vi "Periodic Tasks.vi"(8 "error in":errorcluster) -> ()   [LabVIEW 2014]
doc: "This VI runs in parallel to other tasks. It can contain as many user-defined periodic loops as you need. These can carry out PID or other sorts of timed response."
uses:
  <vilib>/Rock Robotics/WPI/Joystick/WPI_JoystickGetSetRefNum.vi
  <vilib>/Rock Robotics/WPI/RobotDrive/WPI_RobotDriveGetSetRefNum.vi
  Robot Global Data.vi
  <vilib>/Rock Robotics/WPI/RobotDrive/WPI_RobotDriveMecanumDrive_Cartesian.vi
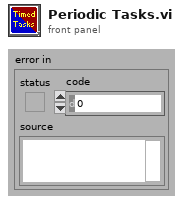
[diagram p1: front panel]
types:
  T1 = typedef "WPI_JoystickDevRef.ctl" = cluster{"Device":T2}
  T2 = typedef "WPI_JoystickDeviceEnum.ctl" = enum16{"USB 0", "USB 1", "USB 2", "USB 3", "USB 4", "USB 5"}
  T3 = typedef "WPI_RobotDriveDevRef.ctl" = cluster{"DevStatus":errorcluster, "Motors[]":T4[], "Square Inputs":bool, "Max Output":dbl}
  T4 = typedef "WPI_MotorControlDeviceRef.ctl" = cluster{"DeviceStatus":errorcluster, "Type":T5, "PWM":cluster{"Controller":T6, "PWM Channel":T7, "DeadBand":T8}, "CAN":cluster{"Device Number":u8, "Control Mode":T9, "Semaphore":T10, "Max Vout":dbl, "TalonSRX Control Mode":T11}, "Invert":bool, "TransformRef":T12, "InvTransformRef":T12}
  T5 = typedef "WPI_MotorControlType.ctl" = enum16{"PWM", "CAN", "CANTalonSRX"}
  T6 = typedef "FPGA_TypedefDigitalModule.ctl" = enum16{"Controller 1"}
  T7 = typedef "FPGA_DIOPWMChannel.ctl" = enum8{"PWM 0", "PWM 1", "PWM 2", "PWM 3", "PWM 4", "PWM 5", "PWM 6", "PWM 7", "PWM 8", "PWM 9", "PWM MXP 0", "PWM MXP 1", "PWM MXP 2", "PWM MXP 3", "PWM MXP 4", "PWM MXP 5", "PWM MXP 6", "PWM MXP 7", "PWM MXP 8", "PWM MXP 9", "Invalid"}
  T8 = typedef "WPI_PWMDeadband.ctl" = cluster{"Name":string, "maxPositivePwm":i32, "minPositivePwm":i32, "centerPwm":i32, "maxNegativePwm":i32, "minNegativePwm":i32, "angularRange":u16}
  T9 = typedef "WPI_CANJaguar_ControlMode.ctl" = enum8{"Percent VBus", "Current", "Speed", "Position", "Voltage"}
  T10 = typedef "Semaphore RefNum" = refnum<k1>
  T11 = typedef "WPI_CANTalonSRX_APIControlMode.ctl" = enum8{"Percent VBus", "Speed", "Position", "Slave", "Unchanged / Invalid"}
  T12 = typedef "WPI_PWMTransform_ConPane.ctl" = refnum<vi>
  T13 = cluster{"JoystickDevRef":T1, "RobotDriveDevRef":T3}
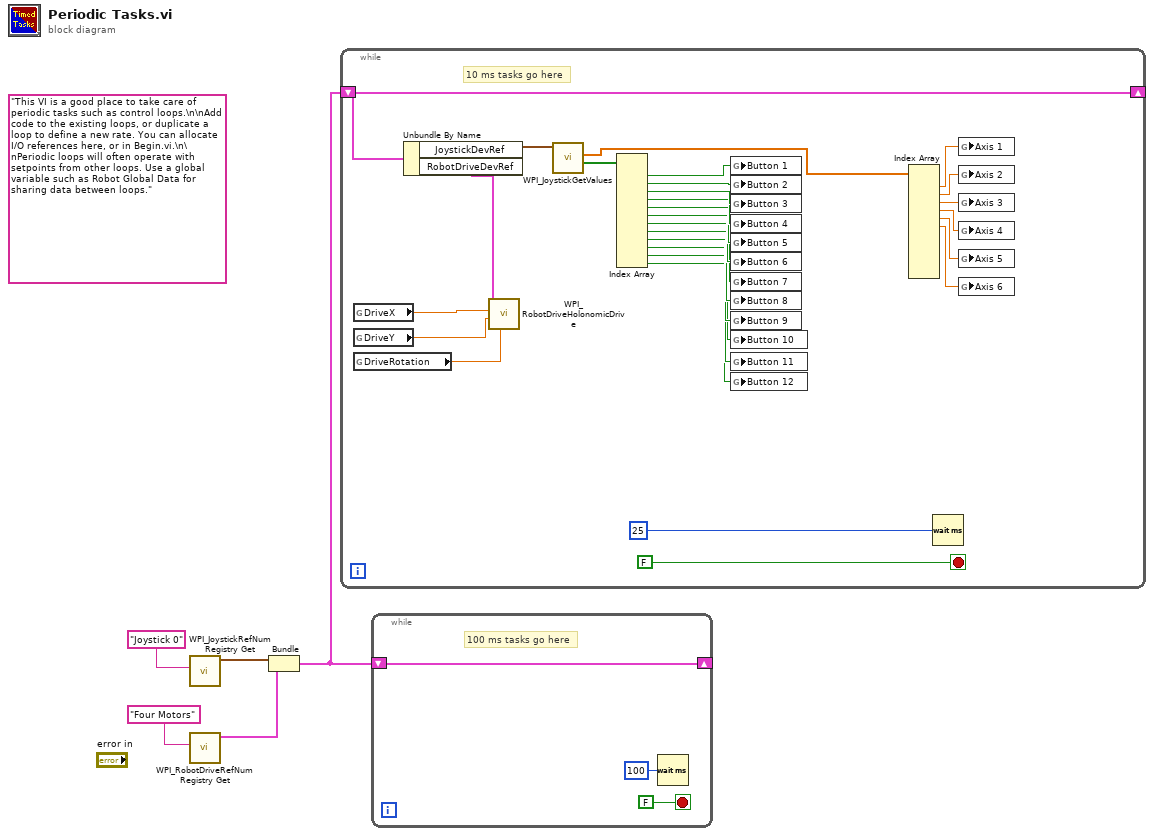
[diagram p0: block diagram]
diagram:
  (unwired) "This VI is a good place to take care of periodic tasks such as control loops.\n\nAdd code to the existing loops, or duplicate a loop to define a new rate. You can allocate I/O references here, or in Begin.vi.\n\nPeriodic loops will often operate with setpoints from other loops. Use a global variable such as Robot Global Data for sharing data between loops."
  n1 = call <vilib>:"WPI_JoystickRefNum Registry Get.vi"("refnum name"="Joystick 0") -> ("JoystickDevRef"=w3:T1)  [unwired: 1 in, 9 out]
  n2 = call <vilib>:"WPI_RobotDriveRefNum Registry Get.vi"("refnum name"="Four Motors") -> ("RobotDriveDevRef"=w2:T3)  [unwired: 1 in, 9 out]
  n3 = Bundle("JoystickDevRef"=w3, "RobotDriveDevRef"=w2) -> (w1:T13)  [unwired: 1 out]
  n4 = while {
    shift-right: [w31] -> _
    shift-left: w1 -> [w31]
    stop <- FALSE stop-if-true
    # "10 ms tasks go here"
    n5 = global read "Robot Global Data.vi" "DriveX"() -> (w8:dbl)
    n6 = global read "Robot Global Data.vi" "DriveY"() -> (w7:dbl)
    n7 = global read "Robot Global Data.vi" "DriveRotation"() -> (w6:dbl)
    n8 = Unbundle By Name(w31) -> ("JoystickDevRef"=w30:T1, "RobotDriveDevRef"=w9:T3)
    n9 = call-poly <vilib>:"WPI_RobotDriveHolonomicDrive.vi"("Rotation"=w6, "Y"=w7, "X"=w8, "RobotDriveDevRef"=w9) -> ()  [unwired: 5 in, 3 out]
    n10 = call <vilib>:"WPI_JoystickGetValues.vi"("JoystickDevRef"=w30) -> ("Buttons"=w29:bool[], "Axes"=w10:dbl[])  [unwired: 6 in, 3 out]
    n11 = Index Array(array=w29) -> (element #1=w28:bool, element #2=w27:bool, element #3=w26:bool, element #4=w25:bool, element #5=w24:bool, element #6=w23:bool, element #7=w22:bool, element #8=w21:bool, element #9=w20:bool, element #10=w19:bool, element #11=w18:bool, element #12=w17:bool)  [unwired: 12 in]
    n12 = global write "Robot Global Data.vi" "Button 1"(w28) -> ()
    n13 = global write "Robot Global Data.vi" "Button 2"(w27) -> ()
    n14 = global write "Robot Global Data.vi" "Button 3"(w26) -> ()
    n15 = global write "Robot Global Data.vi" "Button 4"(w25) -> ()
    n16 = global write "Robot Global Data.vi" "Button 5"(w24) -> ()
    n17 = global write "Robot Global Data.vi" "Button 6"(w23) -> ()
    n18 = global write "Robot Global Data.vi" "Button 7"(w22) -> ()
    n19 = global write "Robot Global Data.vi" "Button 8"(w21) -> ()
    n20 = global write "Robot Global Data.vi" "Button 9"(w20) -> ()
    n21 = global write "Robot Global Data.vi" "Button 10"(w19) -> ()
    n22 = global write "Robot Global Data.vi" "Button 11"(w18) -> ()
    n23 = global write "Robot Global Data.vi" "Button 12"(w17) -> ()
    n24 = Index Array(array=w10) -> (element #1=w16:dbl, element #2=w15:dbl, element #3=w14:dbl, element #4=w13:dbl, element #5=w12:dbl, element #6=w11:dbl)  [unwired: 12 in, 6 out]
    n25 = Wait (ms)(milliseconds to wait=u32 25) -> ()  [unwired: 1 out]
    n26 = global write "Robot Global Data.vi" "Axis 1"(w16) -> ()
    n27 = global write "Robot Global Data.vi" "Axis 2"(w15) -> ()
    n28 = global write "Robot Global Data.vi" "Axis 3"(w14) -> ()
    n29 = global write "Robot Global Data.vi" "Axis 4"(w13) -> ()
    n30 = global write "Robot Global Data.vi" "Axis 5"(w12) -> ()
    n31 = global write "Robot Global Data.vi" "Axis 6"(w11) -> ()
  }
  n32 = while {
    shift-right: [w34] -> _
    shift-left: w1 -> [w34]
    stop <- FALSE stop-if-true
    # "100 ms tasks go here"
    n33 = Wait (ms)(milliseconds to wait=u32 100) -> ()  [unwired: 1 out]
  }
